vi "RandomishWalk.vi"(0 "Y":dbl, 1 "X":dbl, 2 "Max Radius":dbl, 3 "Default Rudder":dbl=9.0, 4 "Alt Rudder":dbl=10.0) -> (5 "Rudder Command":dbl)   [LabVIEW 2012]
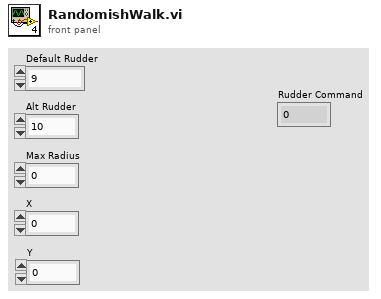
[diagram p1: front panel]
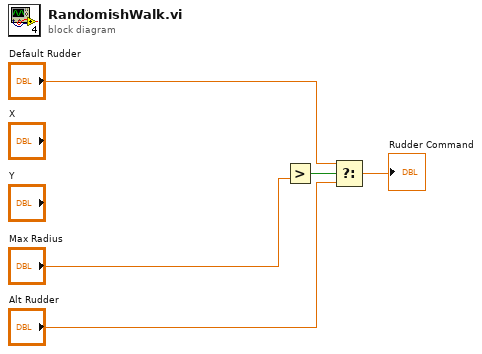
[diagram p0: block diagram]
diagram:
  n1 = Greater?(y="Max Radius") -> (0:w3:bool)  [unwired: 1 in]
  n2 = Select(t="Default Rudder", s=w3, f="Alt Rudder") -> (s? t:f=→"Rudder Command":dbl)
